vi "HMI_GetTestInfoApp.vi"(10 "Mode":enum16{"read", "write"}(ring)=enum."write", 11 "RegTestInfo In":T1) -> (3 "RegTestInfo Out":T1)   [LabVIEW 2024]
uses:
  Control Definitions/DEF_RegTestInfo.ctl
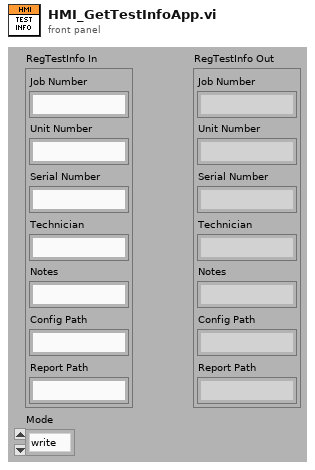
[diagram p1: front panel]
types:
  T1 = typedef "DEF_RegTestInfo.ctl" = cluster{"Job Number":string, "Unit Number":string, "Serial Number":string, "Technician":string, "Notes":string, "Config Path":string, "Report Path":string}
  T2 = cluster{"Key Value out[0]":string, "Key Value out[1]":string, "Key Value out[2]":string, "Key Value out[3]":string, "Key Value out[4]":string, "Key Value out[5]":string, "Key Value out[6]":string}
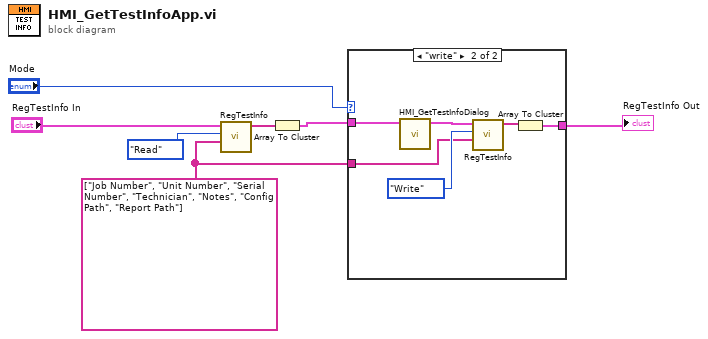
[diagram p0: block diagram]
diagram:
  w3 = string[] ["Job Number", "Unit Number", "Serial Number", "Technician", "Notes", "Config Path", "Report Path"] ("Array")
  n1 = call "RegTestInfo.vi"("Key Definitions"=w3, "Mode"=enum16{"Write", "Read", "Delete"}."Read", "Key Value In"="RegTestInfo In") -> ("Key Value out"=w6:string[])  [unwired: 8 in]
  n2 = Array To Cluster(array=w6) -> (cluster=w4:T2)
  n3 = case shown="\"write\"" "Mode" {
    tunnel: w4 -> [w8 w14]
    tunnel: w3 -> [_ w11]
    tunnel: [w8 w9] -> w1
    frame "read", Default {
    }
    frame "write" {
      n4 = call "HMI_GetTestInfoDialog.vi"("RegTestInfo IN"=w14) -> ("RegTestInfo Out"=w12:T1)  [unwired: 10 in]
      n5 = call "RegTestInfo.vi"("Key Definitions"=w11, "Mode"=enum16{"Write", "Read", "Delete"}."Write", "Key Value In"=w12) -> ("Key Value out"=w10:string[])  [unwired: 8 in]
      n6 = Array To Cluster(array=w10) -> (cluster=w9:T2)
    }
  }
  "RegTestInfo Out" <- w1
